vi "ExSubNframeCol_new_recoveryTRYFIX.vi"(8 "error in (no error)":errorcluster, 9 "image handles":u32[](array[numeric]), 10 "Number of Images":u32=1 min=1 step=1, 11 "Handle Cluster 2":T1) -> (0 "error out":errorcluster, 1 "data handles":u32[](array[numeric]), 2 "x/y":dbl, 3 "Handle Cluster":T1, 4 "x > y?":bool, 6 "image #":i32)   [LabVIEW 2015]
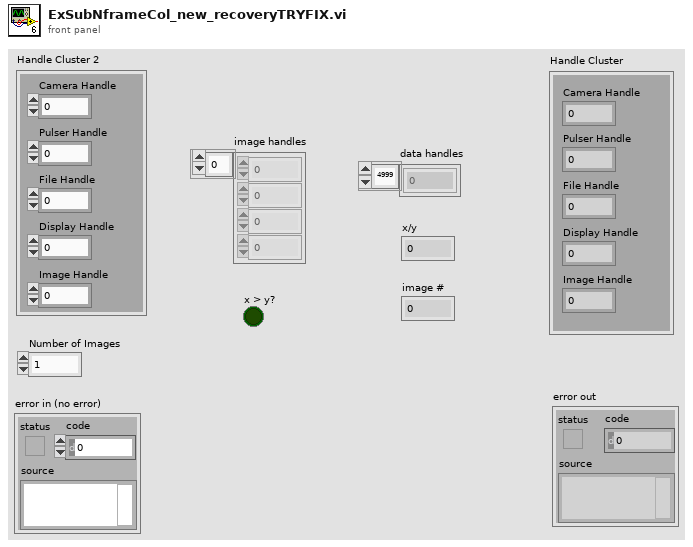
[diagram p1: front panel]
types:
  T1 = cluster{"Camera Handle":u32, "Pulser Handle":u32, "File Handle":u32, "Display Handle":u32, "Image Handle":u32}
  T2 = cluster{"Camera Handle":u32, "Pulser Handle":u32, "File Handle":u32, "Display Handle":u32, "Data Handle":u32}
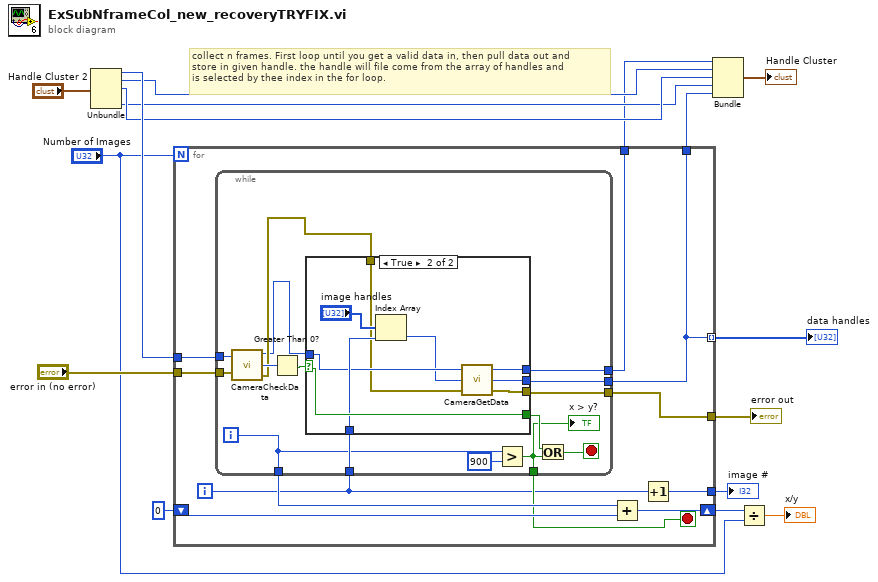
[diagram p0: block diagram]
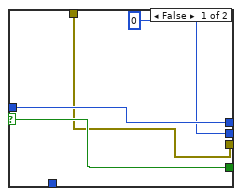
[diagram p2: hidden frame]
diagram:
  # "collect n frames. First loop until you get a valid data in, then pull data out and \nstore in given handle. the handle will file come from the array of handles and\nis selected by thee index in the for loop."
  n1 = Unbundle("Handle Cluster 2") -> ("Camera Handle"=w16:u32, "Pulser Handle"=w13:u32, "File Handle"=w12:u32, "Display Handle"=w11:u32)  [unwired: 1 out]
  n2 = for {
    N: "Number of Images" -> [_]
    tunnel: w16 -> [w27]
    tunnel: "error in (no error)" -> [w26]
    tunnel: [w25] -> w14
    tunnel: [w24] -> w8
    tunnel: [w23] -> w10
    tunnel: [w23] -> w9 mode=indexing
    shift-right: [w22] -> w4
    shift-left: 0 -> [w20]
    tunnel: [w17] -> w1
    i -> [w18]
    stop <- w19 stop-if-true
    n3 = while {
      tunnel: w26 -> [w36]
      tunnel: w27 -> [w37]
      tunnel: [w42] -> w25
      tunnel: w18 -> [w41]
      tunnel: [w40] -> w24
      tunnel: [w39] -> w23
      tunnel: [w30] -> w21
      tunnel: [w31] -> w19
      i -> [w30]
      stop <- w33 stop-if-true
      n4 = call <userlib>:"CameraCheckData.vi"("Camera Handle"=w37, "error in"=w36) -> ("Camera Handle"=w28:u32, "Number Of Frames Available"=w35:i32, "error out"=w29:errorcluster)
      n5 = Greater Than 0?(x=w35) -> (x > 0?=w38:bool)
      n6 = case shown="True" w38 {
        selector: w38 -> [w46 w55]
        tunnel: w28 -> [w45 w52]
        tunnel: [w46 w55] -> w34
        tunnel: [w43 w48] -> w42
        tunnel: w41 -> [_ w54]
        tunnel: [w45 w50] -> w40
        tunnel: [0 w49] -> w39
        tunnel: w29 -> [w43 w47]
        frame False {
        }
        frame True {
          n7 = Index Array(array="image handles", index=w54) -> (element=w51:u32)
          n8 = call <userlib>:"CameraGetData.vi"("error in"=w47, "Data Handle"=w51, "Camera Handle"=w52) -> ("error out"=w48:errorcluster, "Data Handle"=w49:u32, "Camera Handle"=w50:u32)
        }
      }
      n9 = Greater?(x=w30, y=900) -> (0:w31:bool)
      "x > y?" <- w31
      n10 = Or(x=w34, y=w31) -> (x .or. y?=w33:bool)
    }
    n11 = Add(x=w21, y=w20) -> (x+y=w22:i32)
    n12 = Increment(x=w18) -> (x+1=w17:i32)
  }
  "error out" <- w14
  "data handles" <- w9
  "image #" <- w1
  n13 = Bundle("Camera Handle"=w8, "Pulser Handle"=w13, "File Handle"=w12, "Display Handle"=w11, "Data Handle"=w10) -> (→"Handle Cluster":T2)  [unwired: 1 in]
  n14 = Divide(x=w4, y="Number of Images") -> (x/y=→"x/y":dbl)
